vi "Read Serial.vi"(8 "error in":errorcluster, 11 "Base Software in":refnum<class "Main.lvclass">) -> (0 "error out":errorcluster, 2 "Serial":string, 3 "Base Software out":refnum<class "Main.lvclass">)   [LabVIEW 2023, in "Main.lvlib" / "Main.lvclass"]
uses:
  Project/Main.lvclass
  Project/Main.lvclass/Main.ctl
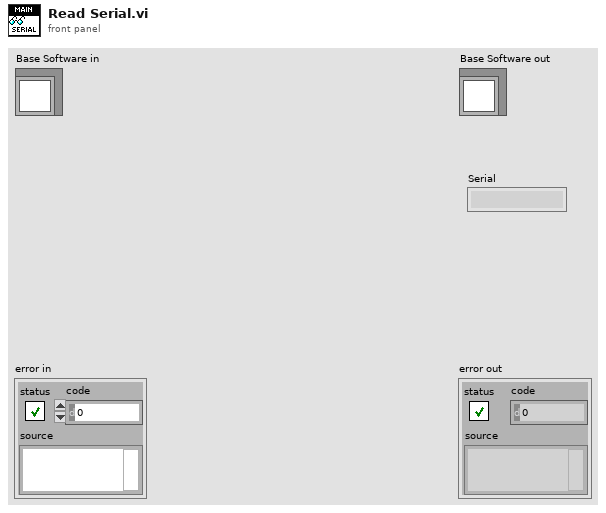
[diagram p1: front panel]
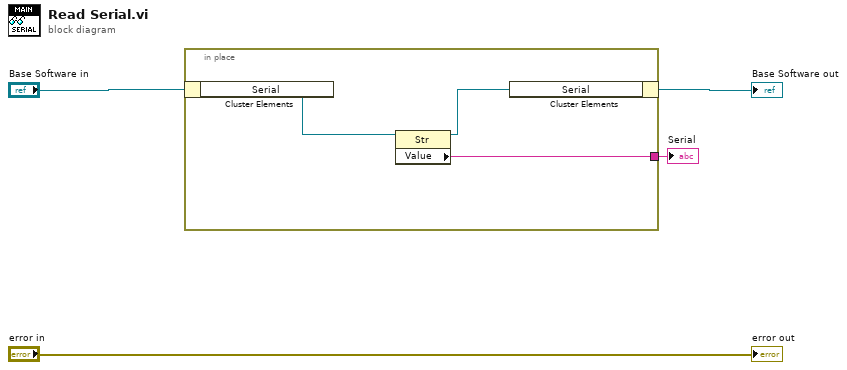
[diagram p0: block diagram]
diagram:
  n1 = in-place {
    in-place-border: [w7] -> w2
    n2 = in-place-cluster #1("Base Software in") -> ("Serial"=w6:refnum<vi>)
    n3 = property class="Str"(reference=w6) -> (reference out=w5:refnum<vi>, "Value"=w7:string)  [unwired: 1 in, 1 out]
    n4 = in-place-cluster #1("Serial"=w5) -> (→"Base Software out":refnum<class "Main.lvclass">)
  }
  "Serial" <- w2
  "error out" <- "error in"
